vi "Read Alicat Data.vi"(8 "error in (no error)":errorcluster, 11 "tCRD Data in":refnum<class "Open Path Data.lvclass">) -> (0 "error out":errorcluster, 2 "Alicat Data":refnum<class "Alicat Data.lvclass">, 3 "tCRD Data out":refnum<class "Open Path Data.lvclass">)   [LabVIEW 2015, in "Open Path Data.lvclass"]
uses:
  Open Path Data.lvclass
  Devices/Alicat/Session Based/Data/Alicat Data.lvclass
  Open Path Data.lvclass/Open Path Data.ctl
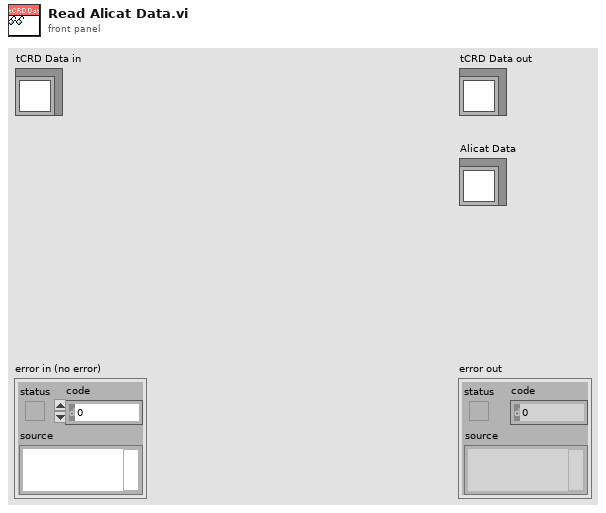
[diagram p1: front panel]
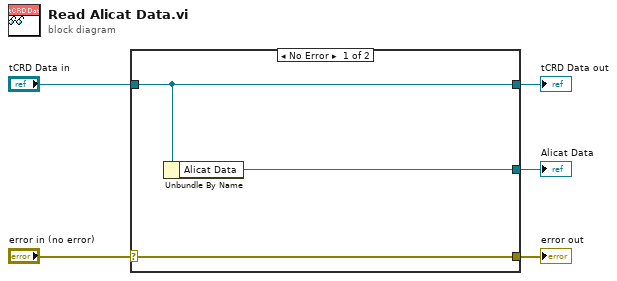
[diagram p0: block diagram]
diagram:
  n1 = case shown="No Error" "error in (no error)" {
    selector: "error in (no error)" -> [w8 w9]
    tunnel: [w8 w9] -> w4
    tunnel: [w7 w10] -> w2
    tunnel: "tCRD Data in" -> [w7 w10]
    tunnel: [w6 _] -> w1
    frame No Error {
      n2 = Unbundle By Name(w7) -> ("Alicat Data"=w6:refnum<class "Alicat Data.lvclass">)
    }
    frame Error {
    }
  }
  "error out" <- w4
  "tCRD Data out" <- w2
  "Alicat Data" <- w1
